vi "example UI get websites.vi"() -> ()   [LabVIEW 2014]
uses:
  dispatcher/execution system.ctl
  dispatcher/pool sizes.ctl
  result/result.lvclass/result.ctl
  result/get data.vi
  result/get data ID.vi
  result/get subresults.vi
  <userlib>/_OpenG.lib/lvdata/lvdata.llb/Get Data Name__ogtk.vi
  <userlib>/_OpenG.lib/error/error.llb/Build Error Cluster__ogtk.vi
  standard action/call by reference action/invoke reentrant method in parallel.vi
  result/result.lvclass
  <vilib>/LAVA/Variant Repository/Write Variant Repository/Write Variant Repository.xnode
  dispatcher/thread pool.lvclass
  standard reporters/event reporter/event reporter.lvclass
  standard action/call by reference action/call function by reference.lvclass
  standard tasks/sequence task/sequence task.lvclass
panel:
  out "websites pulled":i32
  in  "fetch seq":bool
  out "Site data":string
  in  "execution system":T1=enum."other 1"
  in  "fetch par":bool
  in  "Target URLs":string[](array[string])=["www.ni.com/", "www.google.com/", "www.bing.com/", "www.yahoo.com/", "www.microsoft.com/", "www.espn.com/", "www.si.com/", "www.amazon.com/", "www.cnn.com/"]
  in  "Stop":bool
  # "For the code this VI is based on:\nC:\\Program Files (x86)\\National Instruments\\LabVIEW 2013\\examples\\Application Control\\VI Server\\Asynchronous Call By Reference\\Benchmarking Asynchronous Calls.vi"
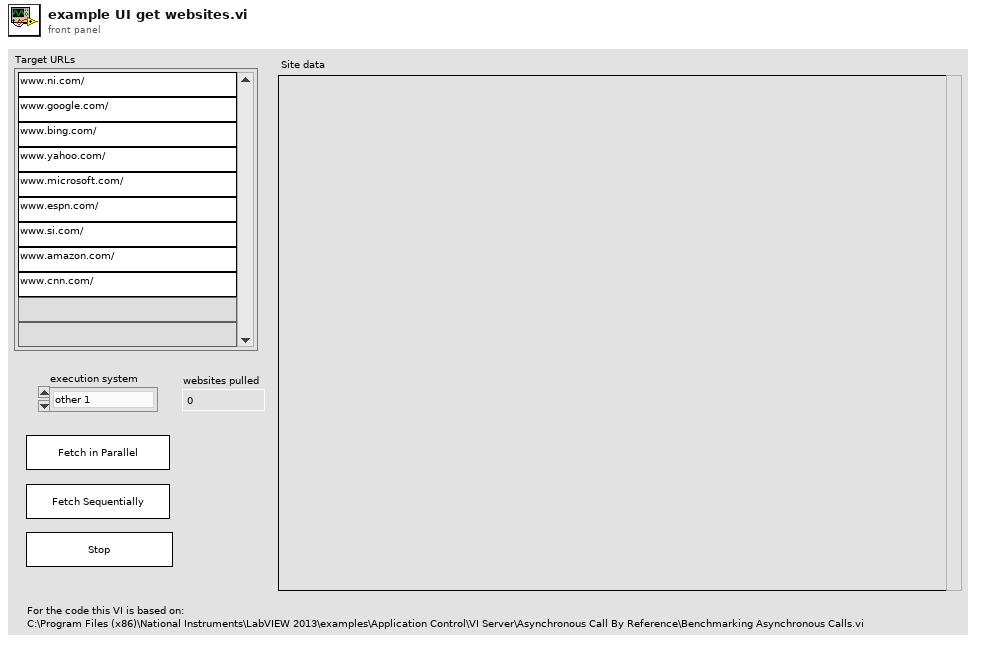
[diagram p1: front panel]
types:
  T1 = typedef "thread pool.lvclass/execution system.ctl" = enum32{"user interface", "standard", "instrument i/o", "data acquisition", "other 1", "other 2"}
  T2 = typedef "thread pool.lvclass/pool sizes.ctl" = cluster{"UI thread":u8, "standard":u8, "instrument I/O":u8, "data acquisition":u8, "other 1":u8, "other 2":u8}
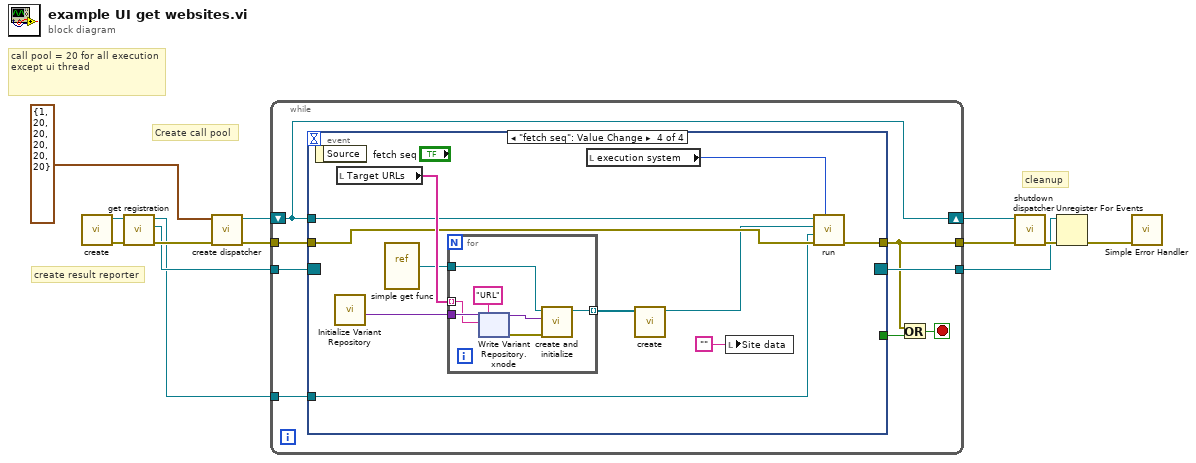
[diagram p0: block diagram]
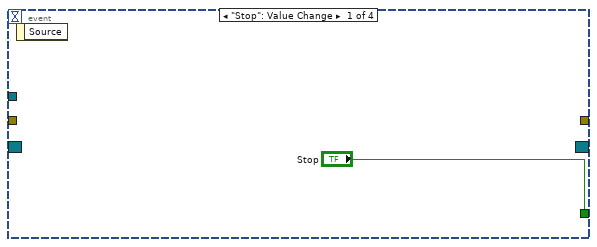
[diagram p2: hidden frame]
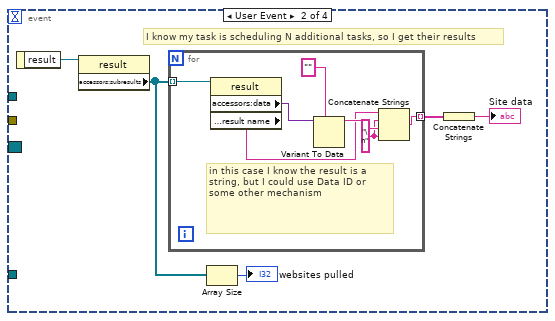
[diagram p3: hidden frame]
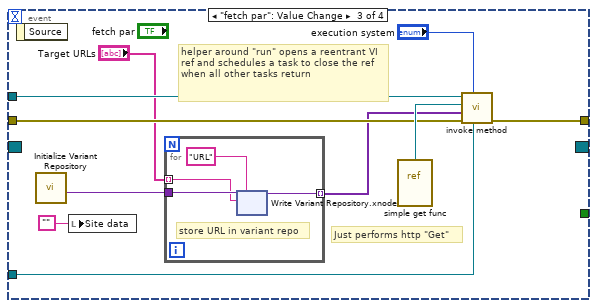
[diagram p4: hidden frame]
diagram:
  # "cleanup"
  # "Create call pool"
  # "call pool = 20 for all execution except ui thread"
  # "create result reporter"
  n1 = call "create.vi"() -> ("error out"=w11:errorcluster, "event reporter out"=w10:refnum<class "event reporter.lvclass">)  [unwired: 10 in]
  n2 = call "get registration.vi"("error in"=w11, "event reporter in"=w10) -> ("error out"=w12:errorcluster, "result registration"=w8:refnum<event-registration>, "event reporter out"=w1:refnum<class "event reporter.lvclass">)  [unwired: 7 in]
  n3 = call "create dispatcher.vi"("error in"=w12, "pool sizes (standard=10)"=T2 {"UI thread"=1, "standard"=20, "instrument I/O"=20, "data acquisition"=20, "other 1"=20, "other 2"=20} ("initial pool sizes")) -> ("error out"=w9:errorcluster, "dispatcher"=w6:refnum<class "thread pool.lvclass">)  [unwired: 8 in]
  n4 = while {
    tunnel: w9 -> [w20]
    tunnel: w8 -> [w19]
    tunnel: [w18] -> w7
    shift-right: [w15] -> w5
    shift-left: w6 -> [w15]
    tunnel: [w16] -> w4
    tunnel: w1 -> [w14]
    stop <- w17 stop-if-true
    n5 = event shown="[3] \"fetch seq\": Value Change" {
      selector: w19 -> [_ _ _ _]
      dyn-events: [_ _ _ _] -> w18
      timeout: _ -> [_ _ _ _]
      tunnel: ["Stop" _ _ _] -> w21
      tunnel: w20 -> [_ _ w43 w117]
      tunnel: [_ _ w42 w116] -> w16
      tunnel: w15 -> [_ _ w41 w115]
      tunnel: w14 -> [_ _ w35 w111]
      event "Stop": Value Change {
        n6 = event-data() -> ()  [unwired: 1 in, 1 out]
      }
      event User Event {
        # "I know my task is scheduling N additional tasks, so I get their results"
        n7 = event-data() -> ("result"=w27:refnum<class "result.lvclass">)  [unwired: 1 in]
        n8 = property class="result"(reference=w27) -> ("accessors:subresults"=w24:refnum<class "result.lvclass">[])  [unwired: 1 in, 2 out]
        n9 = for {
          tunnel: w24 -> [w34] mode=indexing
          tunnel: [w31] -> w26 mode=indexing
          w28 = "\n" ("string")
          # "in this case I know the result is a string, but I could use Data ID or some other mechanism"
          n10 = property class="result"(reference=w34) -> ("accessors:data"=w33:variant, "accessors:result name"=w29:string)  [unwired: 1 in, 2 out]
          n11 = Variant To Data(type="" ("string"), Variant=w33) -> (data=w32:string)  [unwired: 1 in, 1 out]
          n12 = Concatenate Strings(w29, w28, w32, w28) -> (w31:string)
        }
        n13 = Array Size(array=w24) -> (size(s)=→"websites pulled":i32)
        n14 = Concatenate Strings(w26) -> (→"Site data":string)
      }
      event "fetch par": Value Change {
        # "helper around \"run\" opens a reentrant VI ref and schedules a task to close the ref when all other tasks return"
        # "Just performs http \"Get\""
        n15 = event-data() -> ()  [unwired: 1 in, 1 out]
        n16 = call <vilib>:"Initialize Variant Repository.vi"() -> ("Variant Repository"=w40:variant)  [unwired: 11 in]
        n17 = local write "Site data"("") -> ()
        n18 = for {
          tunnel: "Target URLs" -> [w47] mode=indexing
          tunnel: w40 -> [w48]
          tunnel: [w45] -> w38 mode=indexing
          # "store URL in variant repo"
          n19 = xnode "Write Variant Repository.xnode"("Variant Repository In"=w48, "Tag"="URL", "Value"=w47) -> ("Variant Repository Out"=w45:variant)  [unwired: 2 in, 2 out]
        }
        n20 = vi-ref "simple get func.vi"() -> (w44:refnum<vi>)
        n21 = call-poly "invoke method.vi"("results reporter"=w35, "execution system"="execution system", "error in"=w43, "parameters"=w38, "VI in"=w44, "thread pool in"=w41) -> ("error out"=w42:errorcluster)  [unwired: 4 in, 1 out]
      }
      event "fetch seq": Value Change {
        n22 = event-data() -> ()  [unwired: 1 in, 1 out]
        n23 = call <vilib>:"Initialize Variant Repository.vi"() -> ("Variant Repository"=w121:variant)  [unwired: 11 in]
        n24 = local read "Target URLs"() -> (w120:string[])
        n25 = vi-ref "simple get func.vi"() -> (w119:refnum<vi>)
        n26 = for {
          tunnel: w120 -> [w122] mode=indexing
          tunnel: w121 -> [w128]
          tunnel: w119 -> [w124]
          tunnel: [w123] -> w118 mode=indexing
          n27 = xnode "Write Variant Repository.xnode"("Variant Repository In"=w128, "Tag"="URL", "Value"=w122) -> ("Variant Repository Out"=w126:variant, "error out"=w125:errorcluster)  [unwired: 2 in, 1 out]
          n28 = call "create and initialize.vi"("error in"=w125, "parameters"=w126, "function"=w124) -> ("call by reference action"=w123:refnum<class "call function by reference.lvclass">)  [unwired: 7 in, 1 out]
        }
        n29 = local read "execution system"() -> (w112:T1)
        n30 = call "create.vi"("tasks"=w118) -> ("sequence task out"=w114:refnum<class "sequence task.lvclass">)  [unwired: 10 in]
        n31 = local write "Site data"("") -> ()
        n32 = call "run.vi"("execution system"=w112, "error in"=w117, "results reporter"=w111, "task"=w114, "thread pool in"=w115) -> ("error out"=w116:errorcluster)  [unwired: 5 in, 1 out]
      }
    }
    n33 = Or(x=w16, y=w21) -> (x .or. y?=w17:bool)
  }
  n34 = call "shutdown dispatcher.vi"("error in"=w4, "thread pool"=w5) -> ("error out"=w13:errorcluster)  [unwired: 9 in]
  n35 = Unregister For Events(event registration refnum=w7, error in=w13) -> (error out=w2:errorcluster)
  n36 = call <vilib>:"Simple Error Handler.vi"("error in (no error)"=w2) -> ()  [unwired: 4 in, 5 out]
